vi "Affine Transformation.vi"() -> ()   [LabVIEW 2018]
doc: "Affine Transformation: This is an example of affine transformation, which can transform images or geometric shapes in two-dimensional or three-dimensional space through linear transformations and flat transformations. It maintains the original straight lines, parallel lines, and scale relationships in the image."
uses:
  vi.lib/VIRobotics/opencv_yiku/ctls/Point2f.ctl
  vi.lib/VIRobotics/opencv_yiku/ctls/Size.ctl
  vi.lib/VIRobotics/opencv_yiku/Mat/Mat_32F/Mat_32F.lvclass
  D:/Program Files/company/National Instruments/LabVIEW 2018/vi.lib/addons/VIRobotics/opencv_yiku/Mat/Mat/Mat.lvclass
  vi.lib/VIRobotics/opencv_yiku/Mat/Mat_8U/Mat_8U.lvclass
  vi.lib/VIRobotics/opencv_yiku/Mat/Create_Mat_32F.vi
  vi.lib/VIRobotics/opencv_yiku/Cap/Cap.lvclass
  vi.lib/VIRobotics/opencv_yiku/opencv_yiku.lvlib
panel:
  out "new picture 2":picture
  in  "stop":bool
  out "new picture":picture
  # "Overview: Demonstrates how to finish Affine Transformation.\nRequirements: Windows.\nInstructions: \n1.Make sure your computer has a camera.\n2.Run the VI"
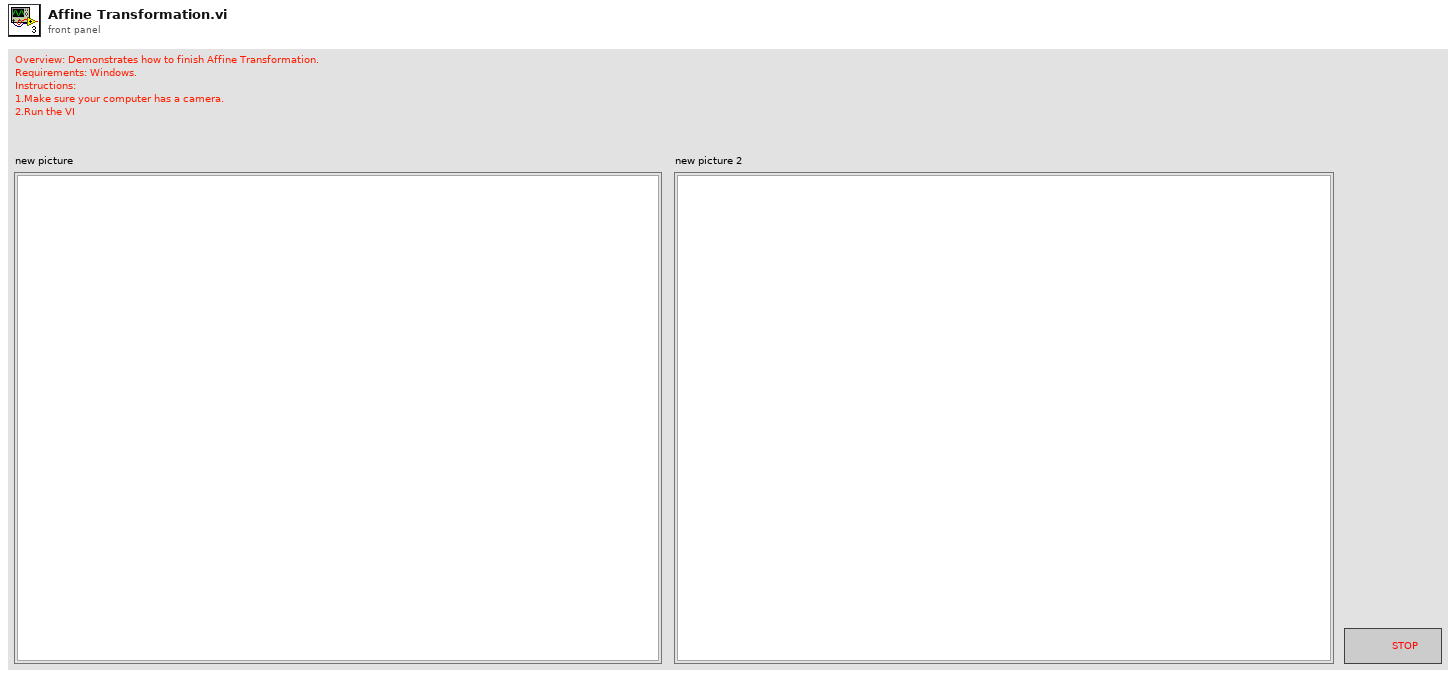
[diagram p1: front panel]
types:
  T1 = typedef "opencv_yiku.lvlib/Point2f.ctl" = cluster{"x":sgl, "y":sgl}
  T2 = typedef "opencv_yiku.lvlib/Size.ctl" = cluster{"x":i32, "y":i32}
  T3 = enum16{"COLOR_BGR2BGRA", "COLOR_BGRA2BGR", "COLOR_BGR2RGBA", "COLOR_RGBA2BGR", "COLOR_BGR2RGB", "COLOR_BGRA2RGBA", "COLOR_BGR2GRAY", "COLOR_RGB2GRAY", "COLOR_GRAY2BGR", "COLOR_GRAY2BGRA"}
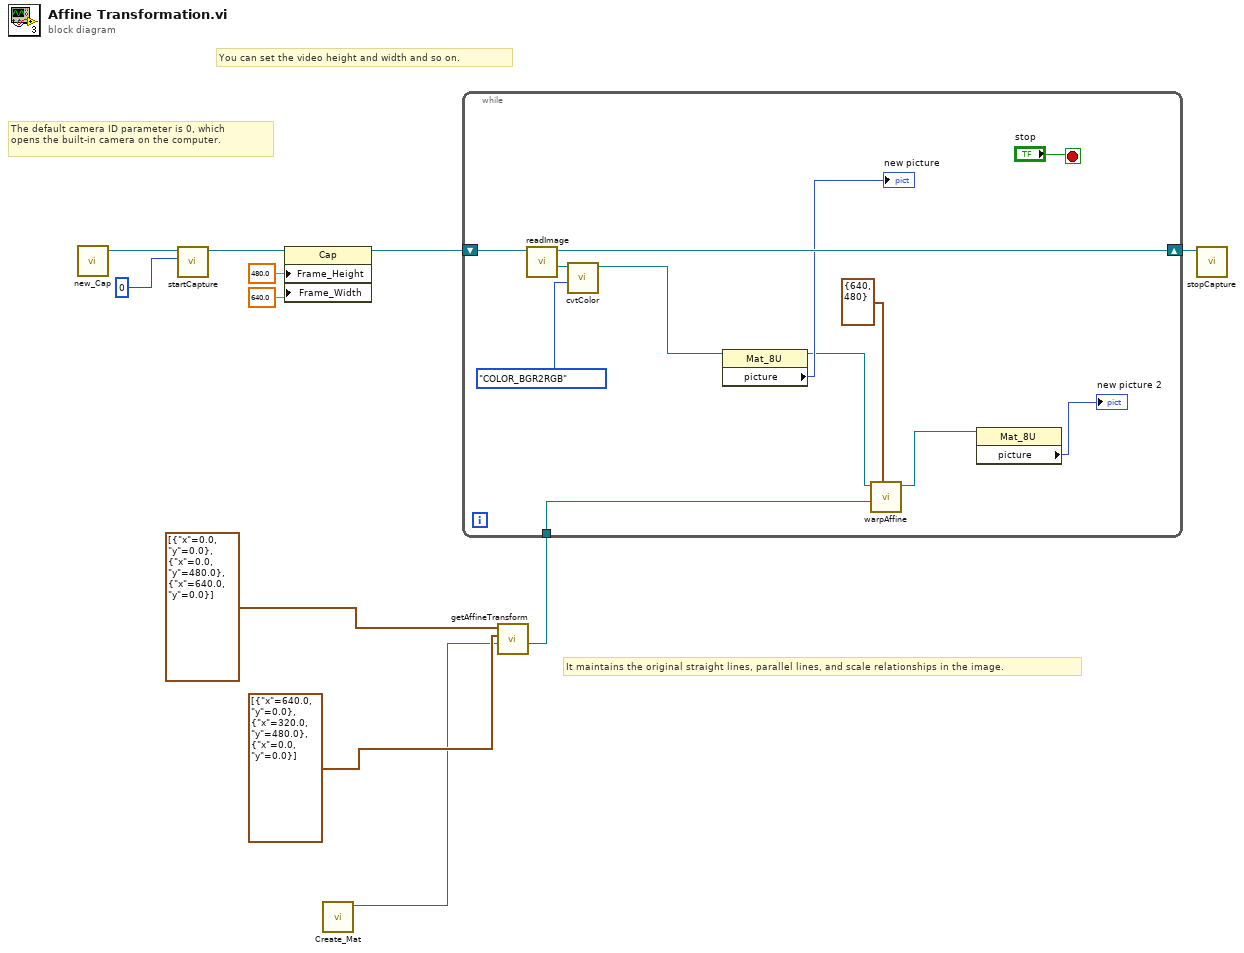
[diagram p0: block diagram]
diagram:
  # "It maintains the original straight lines, parallel lines, and scale relationships in the image."
  # "The default camera ID parameter is 0, which \nopens the built-in camera on the computer."
  # "You can set the video height and width and so on."
  n1 = call "new_Cap.vi"() -> ("Cap out"=w11:refnum<class "Cap.lvclass">)  [unwired: 10 in, 1 out]
  n2 = call "startCapture.vi"("cameraID"=0, "Cap in"=w11) -> ("Cap out"=w8:refnum<class "Cap.lvclass">)  [unwired: 8 in, 1 out]
  n3 = property class="Cap"(reference=w8, "Frame_Height"=480.0, "Frame_Width"=640.0) -> (reference out=w7:refnum<class "Cap.lvclass">)  [unwired: 1 in, 1 out]
  n4 = call-poly "Create_Mat.vi"() -> ("Mat_32F_out"=w2:refnum<class "Mat_32F.lvclass">)  [unwired: 10 in, 1 out]
  n5 = call "getAffineTransform.vi"("Mat"=w2, "dst"=T1[] [{"x"=640.0, "y"=0.0}, {"x"=320.0, "y"=480.0}, {"x"=0.0, "y"=0.0}] ("src"), "src"=T1[] [{"x"=0.0, "y"=0.0}, {"x"=0.0, "y"=480.0}, {"x"=640.0, "y"=0.0}]) -> ("Mat out"=w1:refnum<class "Mat_32F.lvclass">)  [unwired: 7 in, 1 out]
  n6 = while {
    shift-right: [w22] -> w9
    shift-left: w7 -> [w23]
    tunnel: w1 -> [w15]
    stop <- "stop" stop-if-true
    n7 = call "readImage.vi"("Cap in"=w23) -> ("Mat out"=w20:refnum<class "Mat_8U.lvclass">, "Cap out"=w22:refnum<class "Cap.lvclass">)  [unwired: 8 in, 1 out]
    n8 = call "cvtColor.vi"("dstCn"=T3."COLOR_BGR2RGB", "src"=w20) -> ("src out"=w17:refnum<class "Mat_8U.lvclass">)  [unwired: 7 in, 2 out]
    n9 = property class="Mat_8U"(reference=w17) -> (reference out=w16:refnum<class "Mat_8U.lvclass">, "picture"=→"new picture":picture)  [unwired: 1 in, 1 out]
    n10 = call "warpAffine.vi"("Size"=T2 {"x"=640, "y"=480}, "M"=w15, "Mat in"=w16) -> ("dst out"=w13:refnum<class "Mat_8U.lvclass">)  [unwired: 7 in, 1 out]
    n11 = property class="Mat_8U"(reference=w13) -> ("picture"=→"new picture 2":picture)  [unwired: 1 in, 2 out]
  }
  n12 = call "stopCapture.vi"("Cap in"=w9) -> ()  [unwired: 10 in, 1 out]
